vi "Calibration Verify Date Query.vi"(8 "error in (no error)":errorcluster, 11 "VISA resource name":refnum<visa-resource-name>="GPIB0::24::INSTR") -> (0 "error out":errorcluster, 2 "Cal Date":string, 3 "VISA resource name out":refnum<visa-resource-name>)   [LabVIEW 2017, in "Keithley 2450.lvlib"]
doc: "This VI queries the calibration verify date."
uses:
  Keithley 2450.lvlib
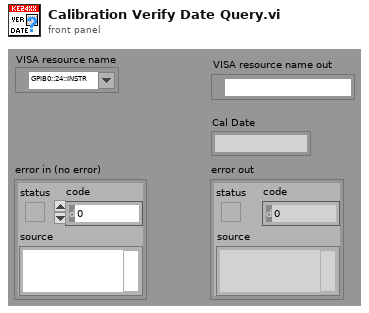
[diagram p1: front panel]
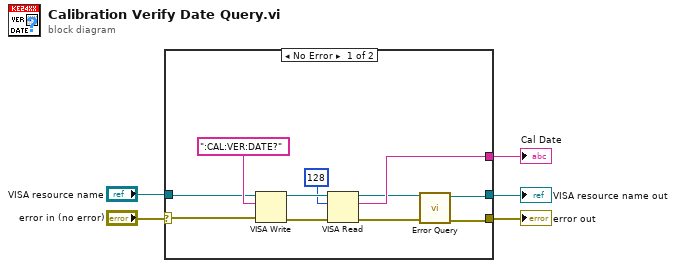
[diagram p0: block diagram]
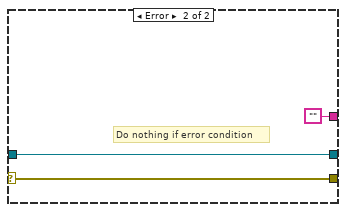
[diagram p2: hidden frame]
diagram:
  n1 = case shown="No Error" "error in (no error)" {
    selector: "error in (no error)" -> [w13 w19]
    tunnel: [w8 w19] -> w4
    tunnel: "VISA resource name" -> [w11 w18]
    tunnel: [w9 w18] -> w2
    tunnel: [w10 "" ("read buffer")] -> w1
    frame No Error {
      n2 = VISA Write(VISA resource name=w11, write buffer=":CAL:VER:DATE?" ("format string"), error in (no error)=w13) -> (VISA resource name out=w15:refnum<visa-resource-name>, error out=w16:errorcluster)  [unwired: 1 out]
      n3 = VISA Read(VISA resource name=w15, byte count=u32 128, error in (no error)=w16) -> (VISA resource name out=w6:refnum<visa-resource-name>, read buffer=w10:string, error out=w7:errorcluster)  [unwired: 1 out]
      n4 = call "Error Query.vi"("error in (no error)"=w7, "VISA resource name"=w6) -> ("error out"=w8:errorcluster, "VISA resource name out"=w9:refnum<visa-resource-name>)  [unwired: 6 in, 2 out]
    }
    frame Error {
      # "Do nothing if error condition"
    }
  }
  "error out" <- w4
  "VISA resource name out" <- w2
  "Cal Date" <- w1
